vi "Teleop.vi"(10 "Match Info":T1={"Autonomous Elapsed Seconds"=0.0, "TeleOp Elapsed Seconds"=0.0, "Disabled Elapsed Seconds"=0.0, "Visited Autonomous"=FALSE, "Visited TeleOp"=FALSE, "Visited Disabled"=FALSE, "Autonomous Settings"={"Autonomous Style"=enum."Independent", "VI Refnum"=refnum}}, 11 "Call Context":T2) -> ()   [LabVIEW 2018]
doc: "This VI is called for each TeleOp packet received from the DS where the robot is not disabled. It is often used to read from the joysticks and update I/O or to update setpoints for timed control loops. It should complete and return within 20 milliseconds or it may miss DS packets."
uses:
  <vilib>/Rock Robotics/WPI/DriverStation/WPI_DriverStationDerivedRobotMode.ctl
  <vilib>/Rock Robotics/WPI/DriverStation/WPI_DriverStationMatch Info.ctl
  <vilib>/Rock Robotics/WPI/Utilities/WPI_GetSetVariantRefNum.vi
  <vilib>/Rock Robotics/Network Tables/NT Write Numeric Array.vi
  MyGlobal.vi
  <vilib>/Rock Robotics/Network Tables/NT Write Boolean Array.vi
panel:
  out "+ pov":dbl
  out "Axe Y":dbl
  out "Axe X":dbl
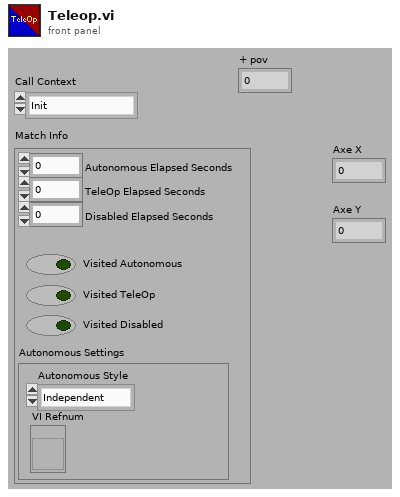
[diagram p1: front panel]
types:
  T1 = typedef "WPI_DriverStationMatch Info.ctl" = cluster{"Autonomous Elapsed Seconds":dbl, "TeleOp Elapsed Seconds":dbl, "Disabled Elapsed Seconds":dbl, "Visited Autonomous":bool, "Visited TeleOp":bool, "Visited Disabled":bool, "Autonomous Settings":cluster{"Autonomous Style":enum16{"Iterative", "Independent"}, "VI Refnum":refnum<vi>}}
  T2 = typedef "WPI_DriverStationDerivedRobotMode.ctl" = enum16{"Init", "Execute", "Stop"}
  T3 = typedef "WPI_JoystickDevRef.ctl" = cluster{"Device":T4}
  T4 = typedef "WPI_JoystickDeviceEnum.ctl" = enum16{"USB 0", "USB 1", "USB 2", "USB 3", "USB 4", "USB 5"}
  T5 = typedef "SwerveDrive.ctl" = cluster{"AVD":cluster{"Angle":dbl, "Vitesse":dbl}, "AVG":cluster{"Angle":dbl, "Vitesse":dbl}, "ARG":cluster{"Angle":dbl, "Vitesse":dbl}, "ARD":cluster{"Angle":dbl, "Vitesse":dbl}}
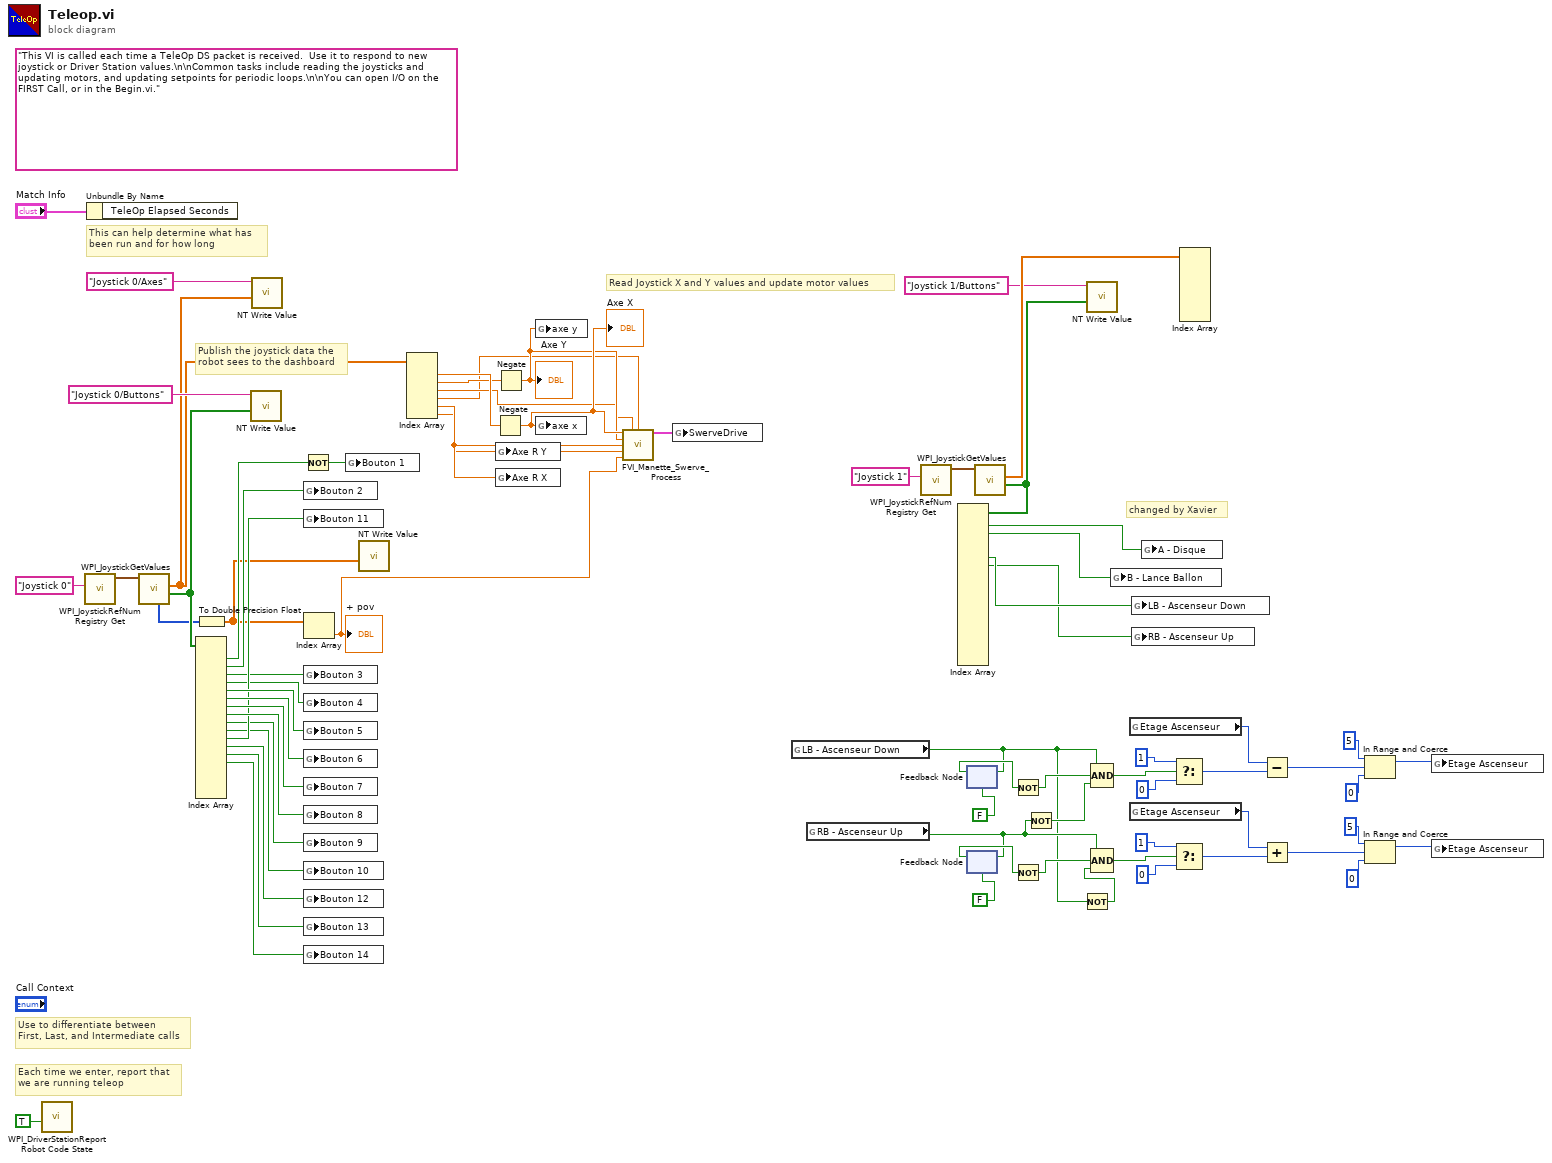
[diagram p0: block diagram]
diagram:
  (unwired) "This VI is called each time a TeleOp DS packet is received.  Use it to respond to new joystick or Driver Station values.\n\nCommon tasks include reading the joysticks and updating motors, and updating setpoints for periodic loops.\n\nYou can open I/O on the FIRST Call, or in the Begin.vi."
  # "changed by Xavier"
  # "Publish the joystick data the\nrobot sees to the dashboard"
  # "Each time we enter, report that\nwe are running teleop"
  # "Use to differentiate between\nFirst, Last, and Intermediate calls"
  # "This can help determine what has\nbeen run and for how long"
  # "Read Joystick X and Y values and update motor values"
  n1 = call <vilib>:"WPI_DriverStationReport Robot Code State.vi"("TeleOp"=TRUE ("Autonomous")) -> ()  [unwired: 10 in, 1 out]
  n2 = call <vilib>:"WPI_JoystickRefNum Registry Get.vi"("refnum name"="Joystick 0") -> ("JoystickDevRef"=w70:T3)  [unwired: 1 in, 9 out]
  n3 = Unbundle By Name("Match Info") -> ()  [unwired: 1 out]
  n4 = call <vilib>:"WPI_JoystickGetValues.vi"("JoystickDevRef"=w70) -> ("Buttons"=w65:bool[], "Axes"=w66:dbl[], "POVs"=w47:i16[])  [unwired: 6 in, 2 out]
  n5 = Index Array(array=w65) -> (element #1=w62:bool, element #2=w52:bool, element #3=w55:bool, element #4=w51:bool, element #5=w60:bool, element #6=w61:bool, element #7=w59:bool, element #8=w58:bool, element #9=w53:bool, element #10=w56:bool, element #11=w57:bool, element #12=w54:bool, element #13=w50:bool, element #14=w49:bool)  [unwired: 18 in, 4 out]
  n6 = To Double Precision Float(number=w47) -> (double precision float=w46:dbl[])
  n7 = call-poly <vilib>:"NT Write Value.vi"("Boolean Array"=w65, "Name"="Joystick 0/Buttons") -> ()  [unwired: 9 in, 1 out]
  n8 = call-poly <vilib>:"NT Write Value.vi"("Numeric Array"=w66, "Name"="Joystick 0/Axes") -> ()  [unwired: 9 in, 1 out]
  n9 = Not(x=w62) -> (.not. x?=w48:bool)
  n10 = global write "MyGlobal.vi" "Bouton 2"(w52) -> ()
  n11 = global write "MyGlobal.vi" "Bouton 11"(w57) -> ()
  n12 = Index Array(array=w46) -> (element=w12:dbl)  [unwired: 1 in]
  "+ pov" <- w12
  n13 = global write "MyGlobal.vi" "Bouton 3"(w55) -> ()
  n14 = global write "MyGlobal.vi" "Bouton 4"(w51) -> ()
  n15 = global write "MyGlobal.vi" "Bouton 5"(w60) -> ()
  n16 = global write "MyGlobal.vi" "Bouton 6"(w61) -> ()
  n17 = global write "MyGlobal.vi" "Bouton 7"(w59) -> ()
  n18 = global write "MyGlobal.vi" "Bouton 8"(w58) -> ()
  n19 = global write "MyGlobal.vi" "Bouton 9"(w53) -> ()
  n20 = global write "MyGlobal.vi" "Bouton 10"(w56) -> ()
  n21 = global write "MyGlobal.vi" "Bouton 12"(w54) -> ()
  n22 = global write "MyGlobal.vi" "Bouton 13"(w50) -> ()
  n23 = global write "MyGlobal.vi" "Bouton 14"(w49) -> ()
  n24 = global write "MyGlobal.vi" "Bouton 1"(w48) -> ()
  n25 = call-poly <vilib>:"NT Write Value.vi"("Numeric Array"=w46) -> ()  [unwired: 10 in, 1 out]
  n26 = Index Array(array=w66) -> (element #1=w64:dbl, element #2=w63:dbl, element #3=w9:dbl, element #4=w8:dbl, element #5=w11:dbl, element #6=w10:dbl)  [unwired: 6 in]
  n27 = Negate(x=w64) -> (-x=w14:dbl)
  "Axe X" <- w14
  n28 = Negate(x=w63) -> (-x=w13:dbl)
  "Axe Y" <- w13
  n29 = global write "MyGlobal.vi" "Axe R Y"(w10) -> ()
  n30 = global write "MyGlobal.vi" "Axe R X"(w11) -> ()
  n31 = global write "MyGlobal.vi" "axe y"(w13) -> ()
  n32 = global write "MyGlobal.vi" "axe x"(w14) -> ()
  n33 = call "FVI_Manette_Swerve_Process.vi"("Axe L X"=w14, "Ltrigger"=w9, "Rtrigger"=w8, "Axe L Y"=w13, "Axe R X"=w11, "Axe R Y"=w10, "POV"=w12) -> ("SwerveDrive"=w45:T5)  [unwired: 8 in]
  n34 = global write "MyGlobal.vi" "SwerveDrive"(w45) -> ()
  n35 = global read "MyGlobal.vi" "LB - Ascenseur Down"() -> (w2:bool)
  n36 = global read "MyGlobal.vi" "RB - Ascenseur Up"() -> (w4:bool)
  n37 = call <vilib>:"WPI_JoystickRefNum Registry Get.vi"("refnum name"="Joystick 1") -> ("JoystickDevRef"=w40:T3)  [unwired: 1 in, 9 out]
  n38 = feedback #1(FALSE) -> (w36:bool)
  n39 = feedback-in #1(w2) -> ()
  n40 = feedback #2(FALSE) -> (w17:bool)
  n41 = feedback-in #2(w4) -> ()
  n42 = call <vilib>:"WPI_JoystickGetValues.vi"("JoystickDevRef"=w40) -> ("Buttons"=w43:bool[], "Axes"=w42:dbl[])  [unwired: 6 in, 3 out]
  n43 = Index Array(array=w43) -> (element #1=w38:bool, element #2=w44:bool, element #5=w7:bool, element #6=w6:bool)  [unwired: 18 in, 14 out]
  n44 = Not(x=w36) -> (.not. x?=w5:bool)
  n45 = Not(x=w17) -> (.not. x?=w16:bool)
  n46 = Not(x=w4) -> (.not. x?=w3:bool)
  n47 = Not(x=w2) -> (.not. x?=w1:bool)
  n48 = call-poly <vilib>:"NT Write Value.vi"("Boolean Array"=w43, "Name"="Joystick 1/Buttons") -> ()  [unwired: 9 in, 1 out]
  n49 = Compound Arithmetic op=AND(w2, w5, w3) -> (w35:bool)
  n50 = Compound Arithmetic op=AND(w4, w16, w1) -> (w18:bool)
  n51 = global write "MyGlobal.vi" "B - Lance Ballon"(w44) -> ()
  n52 = global read "MyGlobal.vi" "Etage Ascenseur"() -> (w31:u8)
  n53 = global read "MyGlobal.vi" "Etage Ascenseur"() -> (w22:u8)
  n54 = global write "MyGlobal.vi" "LB - Ascenseur Down"(w7) -> ()
  n55 = global write "MyGlobal.vi" "RB - Ascenseur Up"(w6) -> ()
  n56 = global write "MyGlobal.vi" "A - Disque"(w38) -> ()
  n57 = Select(t=1, s=w35, f=0) -> (s? t:f=w32:i32)
  n58 = Select(t=1, s=w18, f=0) -> (s? t:f=w21:i32)
  n59 = Index Array(array=w42) -> ()  [unwired: 7 in, 7 out]
  n60 = Subtract(x=w31, y=w32) -> (x-y=w30:i32)
  n61 = Add(x=w22, y=w21) -> (x+y=w23:i32)
  n62 = In Range and Coerce(upper limit=5, x=w30, lower limit=0) -> (coerced(x)=w27:i32)  [unwired: 1 out]
  n63 = In Range and Coerce(upper limit=5, x=w23, lower limit=0) -> (coerced(x)=w26:i32)  [unwired: 1 out]
  n64 = global write "MyGlobal.vi" "Etage Ascenseur"(w27) -> ()
  n65 = global write "MyGlobal.vi" "Etage Ascenseur"(w26) -> ()
